vi "Water Tank Global.vi"() -> ()   [LabVIEW 2013]
panel:
  out "Water level":i32
  out "Bottom":bool
  out "Top":bool
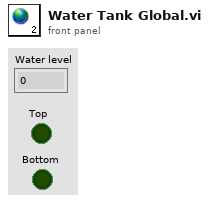
[diagram p1: front panel]
diagram:
